vi "setConfigurationType.vi"(2 "error in (no error)":errorcluster, 3 "Configuration Type":u16(ring)=1 items=["Differential"=10106, "Pseudodifferential"=12529], 4 "niDAQmxAO in":refnum<class "niDAQmxAO.lvclass">) -> (0 "error out":errorcluster, 1 "niDAQmxAO out":refnum<class "niDAQmxAO.lvclass">)   [LabVIEW 2011, in "Hardware.lvlib" / "Channels.lvlib" / "niDAQmxAO.lvclass"]
uses:
  niDAQmxAO.lvclass
  niDAQmxAO.lvclass/niDAQmxAO.ctl
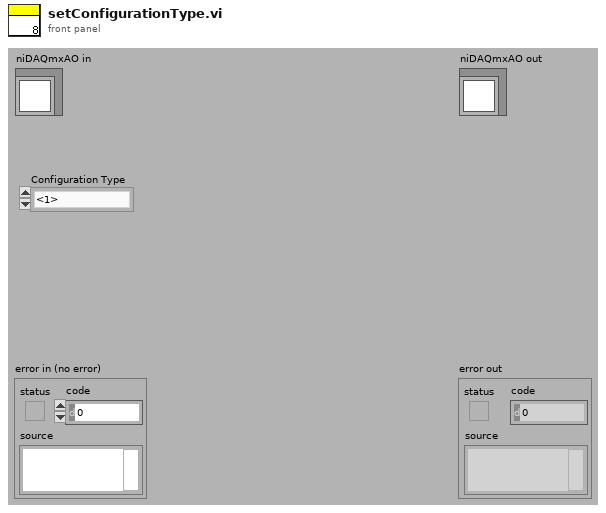
[diagram p1: front panel]
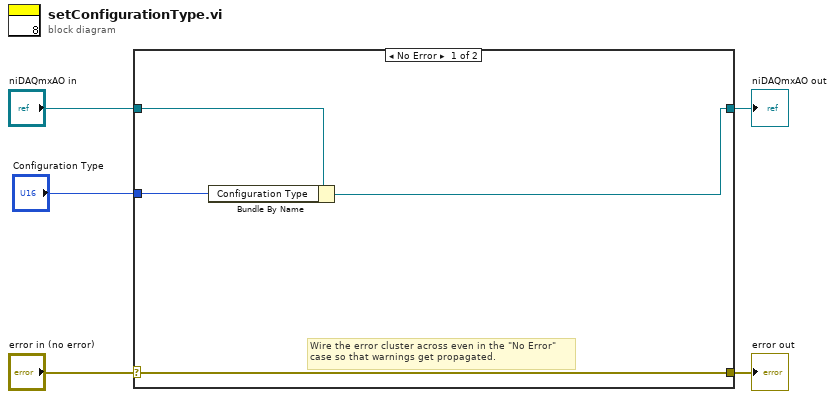
[diagram p0: block diagram]
diagram:
  n1 = case shown="No Error" "error in (no error)" {
    selector: "error in (no error)" -> [w9 w11]
    tunnel: [w9 w11] -> w4
    tunnel: [w7 w10] -> w2
    tunnel: "niDAQmxAO in" -> [w8 w10]
    tunnel: "Configuration Type" -> [w6 _]
    frame No Error {
      # "Wire the error cluster across even in the \"No Error\"\ncase so that warnings get propagated."
      n2 = Bundle By Name(cluster=w8, "Configuration Type"=w6) -> (w7:refnum<class "niDAQmxAO.lvclass">)
    }
    frame Error {
    }
  }
  "error out" <- w4
  "niDAQmxAO out" <- w2
